vi "Test Notifier Synch.vi"() -> ()   [LabVIEW 2021]
uses:
  Source/Support/Nodes/abs_Node/Status.ctl
  Source/System/bt_System.lvclass
  Source/Support/Nodes/Composites/abs_Parallel/Support/Status Calculation.ctl
  Source/Blackboard/Blackboard.lvclass
  Source/Blackboard/Support/Filter Type.ctl
  Source/Support/Nodes/Decorators/Repeater/Support/Finish On - Type.ctl
  Source/Blackboard/Blackboard.lvclass/Blackboard.ctl
  Source/Support/Nodes/Leaves/abs_Type Leaf/abs_Type Leaf.lvclass/abs_Type Leaf.ctl
  Source/Blackboard/Get Value Type/Get I32.vi
  <vilib>/TSA/Abstract Data Classes/Abs_Types/I32 Integer/Static Read.vi
  Source/Blackboard/Support/Index Group.vi
  Source/Blackboard/Support/Index Tags.vi
  Source/Support/Nodes/Leaves/abs_Type Leaf/Properties/Write Value Class.vi
  <vilib>/TSA/Omni-Bus/Local Bus/Support/I32/Local Bus_I32.lvclass
  C:/Program Files (x86)/National Instruments/LabVIEW 2021/vi.lib/TSA/Abstract Data Classes/Abs_Types/Value/Abs_Value.lvclass
  <vilib>/TSA/Abstract Data Classes/Abs_Types/I32 Integer/Abs_I32 Integer.lvclass
  C:/Program Files (x86)/National Instruments/LabVIEW 2021/vi.lib/TSA/Abstract Data Classes/Abs_Types/Numeric/Abs_Numeric.lvclass
  Source/Support/Nodes/Leaves/Test Boolean/Test Abs_Boolean.lvclass
  C:/Users/Tim/Documents/GitHub/LV_Behaviour_Tree/Source/Support/Nodes/abs_Node/bt_Node.lvclass
  C:/Users/Tim/Documents/GitHub/LV_Behaviour_Tree/Source/Support/Nodes/Leaves/abs_Type Leaf/abs_Type Leaf.lvclass
  <vilib>/TSA/Abstract Data Classes/Abs_Types/Boolean/Abs_Boolean.lvclass
  C:/Program Files (x86)/National Instruments/LabVIEW 2021/vi.lib/TSA/Abstract Data Classes/Abs_Types/Type/Abs_Type.lvclass
  <vilib>/TSA/Abstract Data Classes/Constants/Support/I32/I32.vi
  <vilib>/TSA/Omni-Bus/Local Bus/Support/Initialise DVR's.vi
  <vilib>/TSA/Abstract Data Classes/Functions/Math/Support/Increment/I32/Method.vi
  <vilib>/TSA/Abstract Data Classes/Functions/Compare/Support/Greater Equal/I32/Method.vi
  <vilib>/TSA/Abstract Data Classes/Abs_Types/Value/Abs_Value.lvclass
  <vilib>/TSA/Abstract Data Classes/Abs_Types/Type/Abs_Type.lvclass
  <vilib>/TSA/Omni-Bus/Local Bus/Support/DBL/Local Bus_DBL.lvclass
  <vilib>/TSA/Omni-Bus/Local Bus/Support/SGL/Local Bus_SGL.lvclass
  <vilib>/TSA/Omni-Bus/Local Bus/Support/EXT/Local Bus_EXT.lvclass
  <vilib>/TSA/Omni-Bus/Local Bus/Support/Bool/Local Bus_Boolean.lvclass
  <vilib>/TSA/Omni-Bus/Local Bus/Support/STR/Local Bus_String.lvclass
  <vilib>/TSA/Omni-Bus/Local Bus/Support/Variant/Local Bus_Variant.lvclass
  <vilib>/TSA/Omni-Bus/Local Bus/Support/WFM/Local Bus_Waveform.lvclass
  <vilib>/TSA/Omni-Bus/Local Bus/Support/Time/Local Bus_Time.lvclass
  <vilib>/TSA/Omni-Bus/Local Bus/Support/U8/Local Bus_U8.lvclass
  <vilib>/TSA/Omni-Bus/Local Bus/Support/U16/Local Bus_U16.lvclass
  <vilib>/TSA/Omni-Bus/Local Bus/Support/U32/Local Bus_U32.lvclass
  <vilib>/TSA/Omni-Bus/Local Bus/Support/U64/Local Bus_U64.lvclass
  <vilib>/TSA/Omni-Bus/Local Bus/Support/I8/Local Bus_I8.lvclass
  <vilib>/TSA/Omni-Bus/Local Bus/Support/I16/Local Bus_I16.lvclass
  <vilib>/TSA/Omni-Bus/Local Bus/Support/I64/Local Bus_I64.lvclass
  <vilib>/TSA/Omni-Bus/Local Bus/Support/CSGL/Local Bus_CSGL.lvclass
  <vilib>/TSA/Omni-Bus/Local Bus/Support/CDBL/Local Bus_CDBL.lvclass
  <vilib>/TSA/Omni-Bus/Local Bus/Support/CEXT/Local Bus_CEXT.lvclass
  <vilib>/TSA/Omni-Bus/Local Bus/Support/Type/Local Bus_Type.lvclass
  Source/BT.lvlib
  Source/Support/Nodes/Composites/abs_Parallel/bt_Parallel.lvclass
  Source/Support/Nodes/Decorators/Repeater/bt_Repeater.lvclass
  C:/Program Files (x86)/National Instruments/LabVIEW 2021/vi.lib/TSA/Abstract Data Classes/Abs_Types/Integer/Abs_Integer.lvclass
  C:/Program Files (x86)/National Instruments/LabVIEW 2021/vi.lib/TSA/Abstract Data Classes/Abs_Types/I32 Integer/Abs_I32 Integer.lvclass
  <vilib>/TSA/Abstract Data Classes/Functions/Math/Support/Increment/I32/Increment_I32.lvclass
  <vilib>/TSA/Abstract Data Classes/Constants/Support/I32/Const_I32.lvclass
  <vilib>/TSA/Abstract Data Classes/Functions/Compare/Support/Greater Equal/I32/Greater Equal_I32.lvclass
  Source/Support/Nodes/abs_Node/bt_Node.lvclass
panel:
  out "Groups":string[](array[string])
  out "Tags":string[](array[string])
  out "i":u32[](array[numeric])
  out "error out 5":errorcluster
  in  "stop":bool
  out "Status":T1
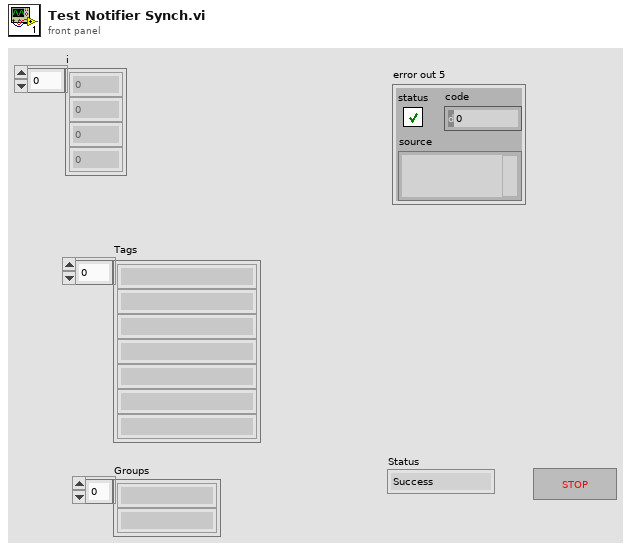
[diagram p1: front panel]
types:
  T1 = typedef "BT.lvlib/bt_Node.lvclass/Status.ctl" = enum16{"Success", "Failure", "Running"}
  T2 = typedef "BT.lvlib/bt_Repeater.lvclass/Finish On - Type.ctl" = enum16{"Success", "Failure", "Never"}
  T3 = typedef "Blackboard.lvclass/Filter Type.ctl" = enum16{"All Tags", "NI Specific Type", "Boolean", "String", "Numeric", "Float", "Integer"}
  T4 = typedef "BT.lvlib/bt_Parallel.lvclass/Status Calculation.ctl" = enum16{"Succeed on All Succeed", "Failure on All Failure", "Succeed on Any Succeed", "Failure on Any Failure"}
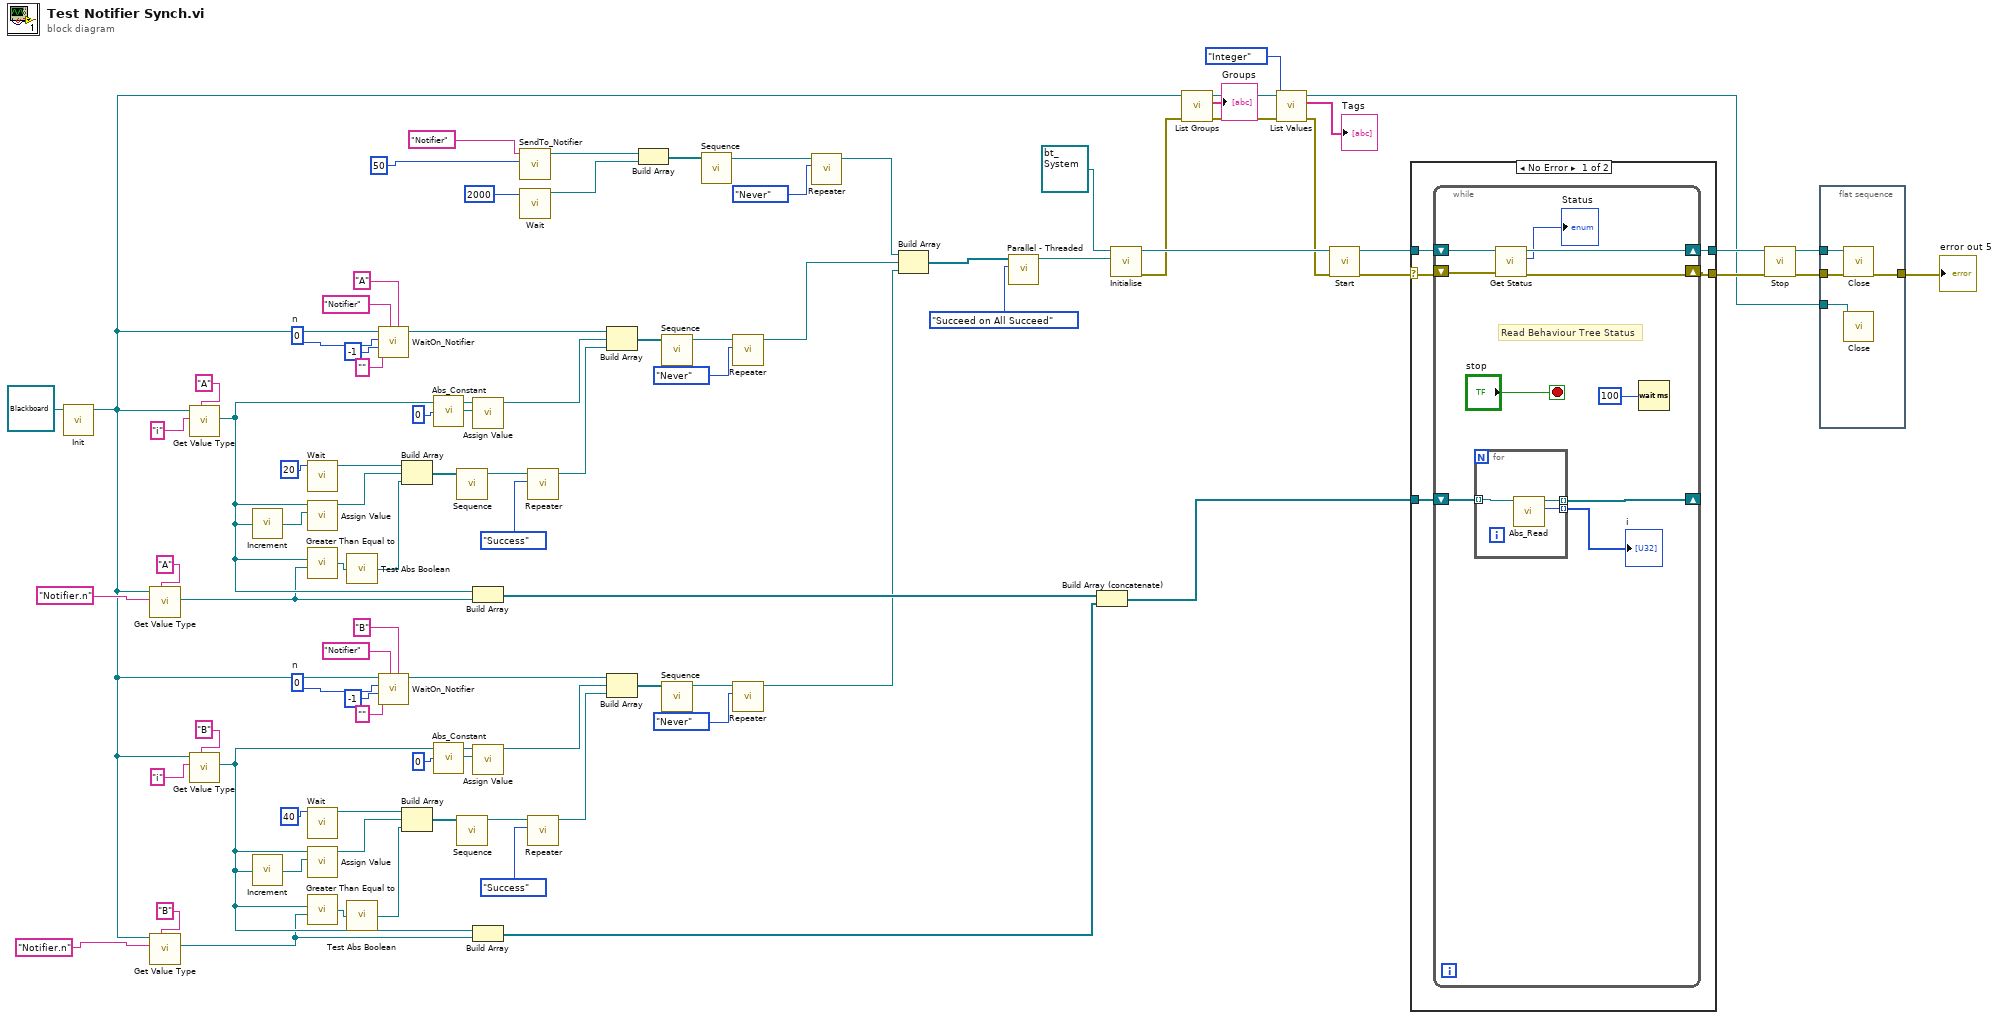
[diagram p0: block diagram]
diagram:
  w27 = 0  # n
  w40 = 0  # n
  n1 = call-dynamic "Init.vi"("bt_Blackboard in"=refnum<class "Blackboard.lvclass"> refnum) -> ("bt_Blackboard out"=w6:refnum<class "Blackboard.lvclass">)  [unwired: 9 in, 1 out]
  n2 = call-poly "Get Value Type.vi"("Tag Group"="A" ("Blackboard Group"), "Tag"="Notifier.n", "Blackboard in"=w6) -> ("Value"=w33:refnum<class "Abs_I32 Integer.lvclass">)  [unwired: 5 in, 3 out]
  n3 = call-poly "Get Value Type.vi"("Tag Group"="B" ("Blackboard Group"), "Tag"="Notifier.n", "Blackboard in"=w6) -> ("Value"=w3:refnum<class "Abs_I32 Integer.lvclass">)  [unwired: 5 in, 3 out]
  n4 = call-poly "Get Value Type.vi"("Tag Group"="A" ("Blackboard Group"), "Tag"="i", "Blackboard in"=w6) -> ("Value"=w58:refnum<class "Abs_I32 Integer.lvclass">)  [unwired: 5 in, 3 out]
  n5 = call-poly "Get Value Type.vi"("Tag Group"="B" ("Blackboard Group"), "Tag"="i", "Blackboard in"=w6) -> ("Value"=w4:refnum<class "Abs_I32 Integer.lvclass">)  [unwired: 5 in, 3 out]
  n6 = call-poly <vilib>:"Increment.vi"("Value"=w58) -> ("Result"=w63:refnum<class "Abs_I32 Integer.lvclass">)  [unwired: 4 in]
  n7 = call-poly <vilib>:"Increment.vi"("Value"=w4) -> ("Result"=w19:refnum<class "Abs_I32 Integer.lvclass">)  [unwired: 4 in]
  n8 = call "Wait.vi"("Time (ms)"=u32 20) -> ("Node Out"=w57:refnum<class "bt_Node.lvclass">)  [unwired: 10 in]
  n9 = call "Assign Value.vi"("Assigned Value"=w63, "Value"=w58) -> ("Node Out"=w62:refnum<class "bt_Node.lvclass">)  [unwired: 9 in]
  n10 = call-poly <vilib>:"Greater Than Equal to.vi"("Value B"=w33, "Value A"=w58) -> ("Result"=w61:refnum<class "Abs_Boolean.lvclass">)  [unwired: 4 in]
  n11 = call "Wait.vi"("Time (ms)"=u32 40) -> ("Node Out"=w24:refnum<class "bt_Node.lvclass">)  [unwired: 10 in]
  n12 = call "Assign Value.vi"("Assigned Value"=w19, "Value"=w4) -> ("Node Out"=w20:refnum<class "bt_Node.lvclass">)  [unwired: 9 in]
  n13 = call-poly <vilib>:"Greater Than Equal to.vi"("Value B"=w3, "Value A"=w4) -> ("Result"=w21:refnum<class "Abs_Boolean.lvclass">)  [unwired: 4 in]
  n14 = call "Test Abs Boolean.vi"("Abs_Boolean.lvclass"=w61) -> ("abs_Node"=w60:refnum<class "bt_Node.lvclass">)  [unwired: 4 in]
  n15 = call "Test Abs Boolean.vi"("Abs_Boolean.lvclass"=w21) -> ("abs_Node"=w22:refnum<class "bt_Node.lvclass">)  [unwired: 4 in]
  n16 = call "WaitOn_Notifier.vi"("Blackboard Group"="A", "Notifier Name"="Notifier" ("Name"), "Tag Root"="", "Timeout (ms)"=-1, "Message Type"=w40, "bt_Blackboard in"=w6) -> ("Node Out"=w39:refnum<class "bt_Node.lvclass">)  [unwired: 4 in, 1 out]
  n17 = call "WaitOn_Notifier.vi"("Blackboard Group"="B", "Notifier Name"="Notifier" ("Name"), "Tag Root"="", "Timeout (ms)"=-1, "Message Type"=w27, "bt_Blackboard in"=w6) -> ("Node Out"=w28:refnum<class "bt_Node.lvclass">)  [unwired: 4 in, 1 out]
  n18 = Build Array(w57, w62, w60) -> (w68:refnum<class "bt_Node.lvclass">[])
  n19 = Build Array(w24, w20, w22) -> (w14:refnum<class "bt_Node.lvclass">[])
  n20 = call-poly <vilib>:"Abs_Constant.vi"("Value"=0 ("n")) -> ("Constant"=w64:refnum<class "Abs_I32 Integer.lvclass">)  [unwired: 4 in]
  n21 = call-poly <vilib>:"Abs_Constant.vi"("Value"=0 ("n")) -> ("Constant"=w18:refnum<class "Abs_I32 Integer.lvclass">)  [unwired: 4 in]
  n22 = call "Sequence.vi"("Nodes"=w68) -> ("Node"=w69:refnum<class "bt_Node.lvclass">)  [unwired: 10 in]
  n23 = call "Sequence.vi"("Nodes"=w14) -> ("Node"=w13:refnum<class "bt_Node.lvclass">)  [unwired: 10 in]
  n24 = call "Assign Value.vi"("Assigned Value"=w64, "Value"=w58) -> ("Node Out"=w59:refnum<class "bt_Node.lvclass">)  [unwired: 9 in]
  n25 = Build Array(w58, w33) -> (w34:refnum<class "Abs_I32 Integer.lvclass">[])
  n26 = call "Assign Value.vi"("Assigned Value"=w18, "Value"=w4) -> ("Node Out"=w23:refnum<class "bt_Node.lvclass">)  [unwired: 9 in]
  n27 = Build Array(w4, w3) -> (w1:refnum<class "Abs_I32 Integer.lvclass">[])
  n28 = call "SendTo_Notifier.vi"("Message"=50, "Queue Name"="Notifier" ("Name")) -> ("Node Out"=w84:refnum<class "bt_Node.lvclass">)  [unwired: 9 in]
  n29 = call "Wait.vi"("Time (ms)"=u32 2000) -> ("Node Out"=w81:refnum<class "bt_Node.lvclass">)  [unwired: 10 in]
  n30 = call "Repeater.vi"("Finish On"=Finish_On_-_Type."Success", "Node In"=w69) -> ("Node Out"=w70:refnum<class "bt_Node.lvclass">)  [unwired: 9 in]
  n31 = call "Repeater.vi"("Finish On"=Finish_On_-_Type."Success", "Node In"=w13) -> ("Node Out"=w12:refnum<class "bt_Node.lvclass">)  [unwired: 9 in]
  n32 = Build Array(w39, w59, w70) -> (w72:refnum<class "bt_Node.lvclass">[])
  n33 = Build Array(w28, w23, w12) -> (w10:refnum<class "bt_Node.lvclass">[])
  n34 = Build Array(w84, w81) -> (w83:refnum<class "bt_Node.lvclass">[])
  n35 = call "Sequence.vi"("Nodes"=w72) -> ("Node"=w71:refnum<class "bt_Node.lvclass">)  [unwired: 10 in]
  n36 = call "Sequence.vi"("Nodes"=w10) -> ("Node"=w11:refnum<class "bt_Node.lvclass">)  [unwired: 10 in]
  n37 = call "Sequence.vi"("Nodes"=w83) -> ("Node"=w43:refnum<class "bt_Node.lvclass">)  [unwired: 10 in]
  n38 = call "Repeater.vi"("Finish On"=Finish_On_-_Type."Never", "Node In"=w71) -> ("Node Out"=w79:refnum<class "bt_Node.lvclass">)  [unwired: 9 in]
  n39 = call "Repeater.vi"("Finish On"=Finish_On_-_Type."Never", "Node In"=w11) -> ("Node Out"=w7:refnum<class "bt_Node.lvclass">)  [unwired: 9 in]
  n40 = call "Repeater.vi"("Finish On"=Finish_On_-_Type."Never", "Node In"=w43) -> ("Node Out"=w42:refnum<class "bt_Node.lvclass">)  [unwired: 9 in]
  n41 = Build Array(w42, w79, w7) -> (w86:refnum<class "bt_Node.lvclass">[])
  n42 = call "Parallel - Threaded.vi"("Status Calculation"=Status_Calculation."Succeed on All Succeed", "Nodes"=w86) -> ("Node"=w85:refnum<class "bt_Node.lvclass">)  [unwired: 9 in]
  n43 = Build Array (concatenate)(w34, w1) -> (w2:refnum<class "Abs_I32 Integer.lvclass">[])
  n44 = call "Initialise.vi"("Behaviour Tree"=w85, "bt_System in"=refnum<class "bt_System.lvclass"> refnum) -> ("error out"=w48:errorcluster, "bt_System out"=w53:refnum<class "bt_System.lvclass">)  [unwired: 8 in]
  n45 = call "List Groups.vi"("error in (no error)"=w48, "Blackboard in"=w6) -> ("error out"=w47:errorcluster, "Groups"=→"Groups":string[], "Blackboard out"=w49:refnum<class "Blackboard.lvclass">)  [unwired: 7 in]
  n46 = call "List Values.vi"("error in (no error)"=w47, "Broad Types"=Filter_Type."Integer", "Blackboard in"=w49) -> ("error out"=w52:errorcluster, "Tags"=→"Tags":string[], "Blackboard out"=w51:refnum<class "Blackboard.lvclass">)  [unwired: 5 in, 1 out]
  n47 = call "Start.vi"("error in (no error)"=w52, "bt_System in"=w53) -> ("error out"=w75:errorcluster, "bt_System out"=w91:refnum<class "bt_System.lvclass">)  [unwired: 8 in]
  n48 = case shown="No Error" w75 {
    selector: w75 -> [w95 w111]
    tunnel: w91 -> [w97 w112]
    tunnel: [w96 w112] -> w88
    tunnel: [w94 w111] -> w73
    tunnel: w2 -> [w93 _]
    frame No Error {
      n49 = while {
        shift-right: [w105] -> w96
        shift-left: w97 -> [w106]
        shift-right: [w101] -> w94
        shift-left: w95 -> [w102]
        shift-right: [w99] -> _
        shift-left: w93 -> [w98]
        stop <- "stop" stop-if-true
        # "Read Behaviour Tree Status"
        n50 = for {
          tunnel: [w110] -> w100 mode=indexing
          tunnel: [w109] -> w99 mode=indexing
          tunnel: w98 -> [w108] mode=indexing
          n51 = call-poly <vilib>:"Abs_Read.vi"("Abs_I32 Integer in"=w108) -> ("Value"=w110:i32, "Abs_I32 Integer out"=w109:refnum<class "Abs_I32 Integer.lvclass">)  [unwired: 8 in, 1 out]
        }
        "i" <- w100
        n52 = call "Get Status.vi"("error in (no error)"=w102, "bt_System in"=w106) -> ("error out"=w101:errorcluster, "Status"=→"Status":T1, "bt_System out"=w105:refnum<class "bt_System.lvclass">)  [unwired: 7 in]
        n53 = Wait (ms)(milliseconds to wait=u32 100) -> ()  [unwired: 1 out]
      }
    }
    frame Error {
    }
  }
  n54 = call "Stop.vi"("error in (no error)"=w73, "bt_System in"=w88) -> ("error out"=w89:errorcluster, "bt_System out"=w90:refnum<class "bt_System.lvclass">)  [unwired: 8 in]
  n55 = flat-sequence {
    tunnel: w90 -> [w116]
    tunnel: w89 -> [w115]
    tunnel: [w114] -> w74
    tunnel: w51 -> [w113]
    frame #0 {
      n56 = call-dynamic "Close.vi"("error in (no error)"=w115, "bt_System in"=w116) -> ("error out"=w114:errorcluster)  [unwired: 8 in, 1 out]
      n57 = call-dynamic "Close.vi"("bt_Blackboard in"=w113) -> ()  [unwired: 9 in, 2 out]
    }
  }
  "error out 5" <- w74
